vi "SensorReadOneLine.vi"() -> ()   [LabVIEW 2016]
uses:
  <vilib>/Instr/_visa.llb/VISA Configure Serial Port (Instr).vi
  Other Models/2010/Status/AxisDiagPacket.ctl
  Other Models/2010/Status/ControllerDiagPacket.ctl
  Control/Coordinate.ctl
panel:
  in  "file (use dialog)":path=path "C:/Users/TTUHEP/Documents/LabVIEW/output.txt"
  out "Boolean":bool=TRUE
  in  "baud rate":u32=115200
  in  "data bits":u16=8 min=5 max=8 step=1
  in  "parity":u16(ring)=2 items=["None", "Odd", "Even", "Mark", "Space"]
  in  "stop bits":u16(ring)=10 items=["1"=10, "1.5"=15, "2.0"=20]
  in  "flow control":u16(ring) items=["None"=0, "XON/XOFF"=1, "RTS/CTS"=2, "DTR/DSR"=4]
  in  "VISA resource name":refnum<visa-resource-name>="COM4"
  in  "Speed":dbl format="%#_13g"
  in  "EndPoint":T1 {"X" format="%#.5g"; "Y" format="%#.5g"; "Z" format="%#.6g"}
  in  "StartPoint":T1 {"X" format="%#.5g"; "Y" format="%#.5g"; "Z" format="%#.5g"}
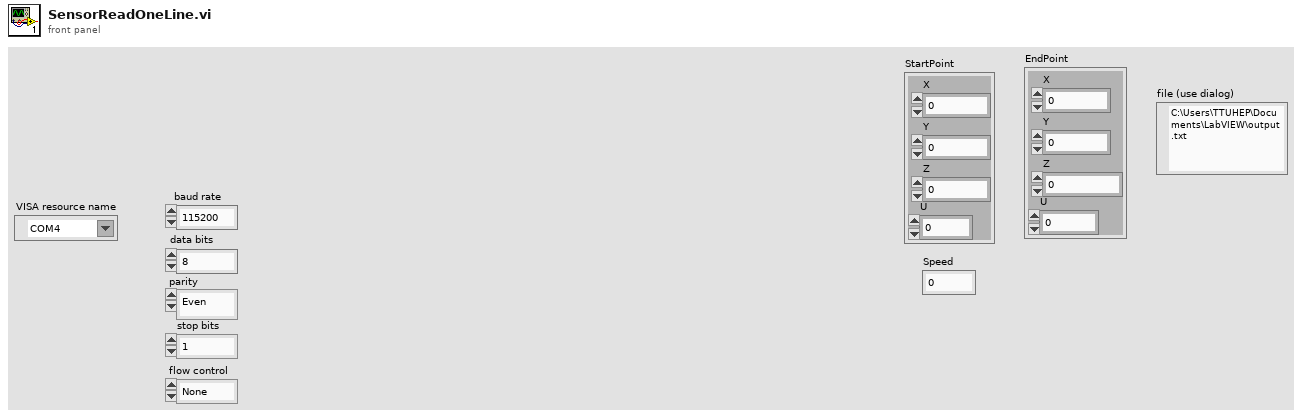
[diagram p1: front panel]
types:
  T1 = typedef "Coordinate.ctl" = cluster{"X":dbl, "Y":dbl, "Z":dbl, "U":dbl}
  T2 = typedef "ControllerDiagPacket.ctl" = cluster{"Number of Diag Packets":i32, "Axes":T3[], "error":errorcluster}
  T3 = typedef "AxisDiagPacket.ctl" = cluster{"Axis Name":string, "Analog Input 0":dbl, "Analog Input 1":dbl, "Axis Fault (num)":i32, "Axis Fault (str)":string, "Axis Fault (bits)":cluster{"AmplifierFault":bool, "AmplifierTemperatureFault":bool, "CcwEndOfTravelLimitFault":bool, "CcwSoftwareLimitFault":bool, "CommunicationLostFault":bool, "CwEndOfTravelLimitFault":bool, "CwSoftwareLimitFault":bool, "EmergencyStopFault":bool, "EncoderFault":bool, "ExternalFault":bool, "FeedbackScalingFault":bool, "GantryMisalignFault ":bool, "HallSensorFault":bool, "InPositionTimeoutFault":bool, "InternalFault":bool, "MarkerSearchFault":bool, "MaxVelocityCommandFault":bool, "MissedInterruptFault":bool, "MotorTemperatureFault":bool, "None":bool, "OverCurrentFault":bool, "PositionErrorFault":bool, "PositionFeedbackFault":bool, "PowerSupplyFault":bool, "ProbeInputFault":bool, "SafeZoneFault":bool, "VelocityErrorFault":bool, "VelocityFeedbackFault":bool, "VoltageClampFault":bool}, "Axis Status (num)":i32, "Axis Status (str)":string, "Axis Status (bits)":cluster{"BacklashActive":bool, "CalibrationEnabled1D":bool, "CalibrationEnabled2D":bool, "CommandValid":bool, "DriveAbortPending":bool, "DrivePending":bool, "Enabling":bool, "GainMappingEnabled":bool, "GantryAligned":bool, "GantryRealigning":bool, "Homed":bool, "Homing":bool, "IFOVEnabled":bool, "JogGenerating":bool, "Jogging":bool, "JoystickControl":bool, "MasterSlaveControl":bool, "MotionBlocked":bool, "MotionClamped":bool, "MoveDone":bool, "None":bool, "NotVirtual":bool, "Profiling":bool, "Stability0":bool, "Stability1":bool, "TrajectoryFiltering":bool, "WaitDone":bool}, "Current Command":sgl, "Current Error":sgl, "Current Feedback":sgl, "Digital Inputs":i32, "Digital Outputs":i32, "Drive Status":i32, "Drive Status (str)":string, "Drive Status (bits)":cluster{"AccelerationPhase":bool, "AutofocusActive":bool, "BrakeOutput":bool, "CcwEndOfTravelLimitInput":bool, "CosineEncoderError":bool, "CurrentClamp":bool, "CwEndOfTravelLimitInput":bool, "DecelerationPhase":bool, "DualLoopActive":bool, "EmergencyStopInput":bool, "Enabled":bool, "EncoderClipping":bool, "GalvoCalibrationEnabled":bool, "GalvoPowerCorrection":bool, "HallAInput":bool, "HallBInput":bool, "HallCInput":bool, "HighResolutionMode":bool, "HomeLimitInput":bool, "InPosition":bool, "InPosition2":bool, "MarkerInput":bool, "MarkerLatch":bool, "MoveActive":bool, "NoMotorSupply":bool, "None":bool, "PowerLimiting":bool, "ProgrammingFlash":bool, "ProgrammingMXH":bool, "PSOHaltLatch":bool, "ServoControl":bool, "SineEncoderError":bool}, "Position Feedback Auxiliary":dbl, "Position Command":dbl, "Position Error":dbl, "Position Feedback":dbl, "Program Position Command":dbl, "Program Position Error":dbl, "Program Position Feedback":dbl, "Velocity Command":dbl, "Velocity Error":dbl, "Velocity Feedback":dbl}
  T4 = cluster{"ControllerDiagPacket":T2, "read buffer":string}
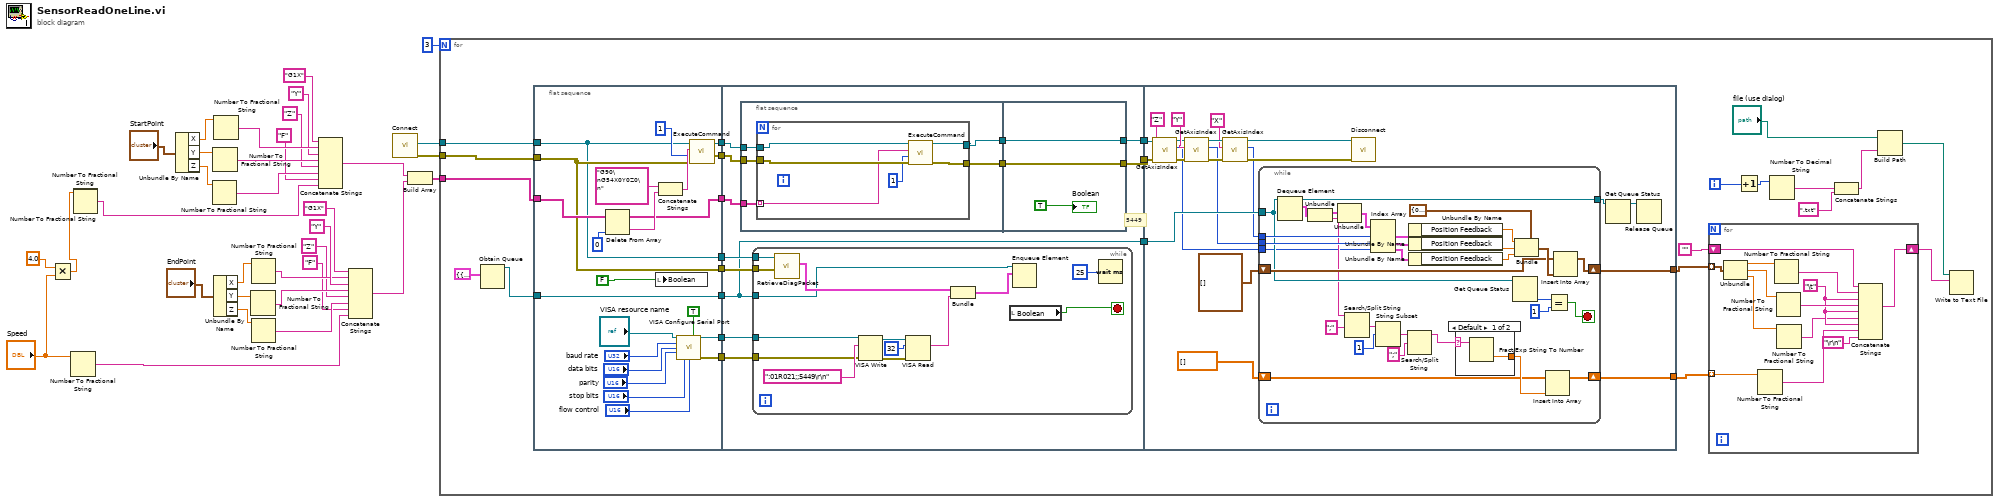
[diagram p0: block diagram]
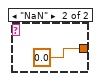
[diagram p2: hidden frame]
diagram:
  n1 = Multiply(x=4.0, y="Speed") -> (x*y=w2:dbl)
  n2 = Number To Fractional String(number="Speed") -> (F-format string=w8:string)  [unwired: 3 in]
  n3 = Number To Fractional String(number=w2) -> (F-format string=w1:string)  [unwired: 3 in]
  n4 = Number To Fractional String() -> ()  [unwired: 4 in, 1 out]
  n5 = Unbundle By Name("StartPoint") -> ("X"=w32:dbl, "Y"=w31:dbl, "Z"=w10:dbl)
  n6 = Number To Fractional String(number=w10) -> (F-format string=w15:string)  [unwired: 3 in]
  n7 = Number To Fractional String(number=w31) -> (F-format string=w29:string)  [unwired: 3 in]
  n8 = Number To Fractional String(number=w32) -> (F-format string=w30:string)  [unwired: 3 in]
  n9 = Unbundle By Name("EndPoint") -> ("X"=w21:dbl, "Y"=w22:dbl, "Z"=w13:dbl)
  n10 = Number To Fractional String(number=w22) -> (F-format string=w24:string)  [unwired: 3 in]
  n11 = Number To Fractional String(number=w21) -> (F-format string=w23:string)  [unwired: 3 in]
  n12 = Number To Fractional String(number=w13) -> (F-format string=w12:string)  [unwired: 3 in]
  n13 = Concatenate Strings("G1X", w30, "Y", w29, "Z", w15, "F", w1) -> (w19:string)
  n14 = Concatenate Strings("G1X", w23, "Y", w24, "Z", w12, "F", w8) -> (w18:string)
  n15 = call "Connect.vi"() -> ("error out"=w7:errorcluster, "controller"=w6:refnum<k24>)  [unwired: 10 in]
  n16 = Build Array(w19, w18) -> (w17:string[])
  n17 = for {
    N: 3 -> [_]
    tunnel: w17 -> [w49]
    tunnel: w7 -> [w42]
    tunnel: w6 -> [w41]
    i -> [w40]
    # "5449"
    n18 = Obtain Queue(element data type=cluster{"ControllerDiagPacket":T2, string} {"ControllerDiagPacket"={"Number of Diag Packets"=0, "Axes"=[], "error"={"status"=FALSE, "code"=0, "source"=""}}, ""}) -> (queue out=w47:refnum<queue>)  [unwired: 4 in, 2 out]
    n19 = flat-sequence {
      tunnel: [w89] -> w60
      tunnel: [w93] -> w59
      tunnel: [w94] -> w58
      tunnel: w49 -> [w95]
      tunnel: [w74] -> w57
      tunnel: [w75] -> w56
      tunnel: w47 -> [w87]
      tunnel: [w87] -> w55
      tunnel: [w79] -> w54
      tunnel: [w78] -> w53
      tunnel: w42 -> [w75]
      tunnel: w41 -> [w74]
      tunnel: [w102] -> w52
      tunnel: w60 -> [w96]
      tunnel: w59 -> [w98]
      tunnel: w58 -> [w97]
      tunnel: w57 -> [w106]
      tunnel: w56 -> [w107]
      tunnel: w55 -> [w105]
      tunnel: [w105] -> w51
      tunnel: w54 -> [w104]
      tunnel: w53 -> [w103]
      tunnel: [w99] -> w50
      tunnel: w52 -> [w141]
      tunnel: w51 -> [w156]
      tunnel: [w143] -> w43
      tunnel: [w142] -> w44
      tunnel: w50 -> [w140]
      frame #0 {
        n20 = Delete From Array(array=w95, index=0) -> (deleted portion=w90:string, array with subset deleted=w89:string[])  [unwired: 1 in]
        n21 = local write "Boolean"(FALSE) -> ()
        n22 = Concatenate Strings("G90\nG54X0Y0Z0\n", w90) -> (w88:string)
        n23 = call-poly "VISA Configure Serial Port"("VISA resource name"="VISA resource name", "Enable Termination\nChar (T)"=TRUE, "baud rate (9600)"="baud rate", "data bits (8)"="data bits", "parity (0:none)"="parity", "stop bits (10: 1 bit)"="stop bits", "flow control (0:none)"="flow control") -> ("VISA resource name out"=w79:refnum<visa-resource-name>, "error out"=w78:errorcluster)  [unwired: 7 in]
        n24 = call "ExecuteCommand.vi"("error in (no error)"=w75, "taskId"=1, "Command Code"=w88, "controller in"=w74) -> ("error out"=w94:errorcluster, "controller out"=w93:refnum<k24>)  [unwired: 5 in, 1 out]
      }
      frame #1 {
        n25 = flat-sequence {
          tunnel: [w112] -> w101
          tunnel: [w111] -> w100
          tunnel: w98 -> [w110]
          tunnel: w97 -> [w109]
          tunnel: w96 -> [w108]
          tunnel: [w120] -> w102
          tunnel: w101 -> [w120]
          tunnel: w100 -> [w119]
          tunnel: [w119] -> w99
          frame #0 {
            n26 = for {
              tunnel: w108 -> [w116] mode=indexing
              tunnel: w110 -> [w117]
              tunnel: w109 -> [w118]
              tunnel: [w114] -> w112
              tunnel: [w113] -> w111
              n27 = call "ExecuteCommand.vi"("error in (no error)"=w118, "taskId"=1, "Command Code"=w116, "controller in"=w117) -> ("error out"=w114:errorcluster, "controller out"=w113:refnum<k24>)  [unwired: 5 in, 1 out]
            }
          }
          frame #1 {
            "Boolean" <- TRUE
          }
        }
        n28 = while {
          tunnel: w106 -> [w135]
          tunnel: w107 -> [w134]
          tunnel: w105 -> [w122]
          tunnel: w104 -> [w131]
          tunnel: w103 -> [w129]
          stop <- w123 stop-if-true
          n29 = call "RetrieveDiagPacket.vi"("error in (no error)"=w134, "Controller In"=w135) -> ("ControllerDiagPacket"=w126:T2)  [unwired: 7 in, 2 out]
          n30 = VISA Write(VISA resource name=w131, write buffer=":01R021;;5449\r\n", error in (no error)=w129) -> (VISA resource name out=w132:refnum<visa-resource-name>, error out=w128:errorcluster)  [unwired: 1 out]
          n31 = VISA Read(VISA resource name=w132, byte count=u32 32, error in (no error)=w128) -> (read buffer=w125:string)  [unwired: 3 out]
          n32 = Bundle("ControllerDiagPacket"=w126, "read buffer"=w125) -> (w124:T4)  [unwired: 1 in]
          n33 = local read "Boolean"() -> (w123:bool)
          n34 = Enqueue Element(queue=w122, element=w124) -> ()  [unwired: 2 in, 3 out]
          n35 = Wait (ms)(milliseconds to wait=25) -> ()  [unwired: 1 out]
        }
      }
      frame #2 {
        n36 = call "GetAxisIndex.vi"("error in (no error)"=w141, "axis name"="Z", "controller in"=w140) -> ("error out"=w138:errorcluster, "axis index"=w136:i32, "controller out"=w139:refnum<k24>)  [unwired: 6 in]
        n37 = call "GetAxisIndex.vi"("error in (no error)"=w138, "axis name"="Y", "controller in"=w139) -> ("error out"=w154:errorcluster, "axis index"=w148:i32, "controller out"=w155:refnum<k24>)  [unwired: 6 in]
        n38 = call "GetAxisIndex.vi"("error in (no error)"=w154, "axis name"="X", "controller in"=w155) -> ("error out"=w153:errorcluster, "axis index"=w149:i32, "controller out"=w152:refnum<k24>)  [unwired: 6 in]
        n39 = while {
          tunnel: w149 -> [w186]
          tunnel: w148 -> [w185]
          shift-right: [w178] -> w142
          shift-left: cluster{"X":dbl, "Y":dbl, "Y 2":dbl}[] [] -> [w176]
          tunnel: [w177] -> w146
          tunnel: w156 -> [w172]
          shift-right: [w160] -> w143
          shift-left: dbl[] [] -> [w161]
          tunnel: w136 -> [w159]
          stop <- w174 stop-if-true
          n40 = Dequeue Element(queue=w172) -> (queue out=w177:refnum<queue>, element=w171:cluster{"ControllerDiagPacket":T2, string})  [unwired: 2 in, 2 out]
          n41 = Unbundle(w171) -> ("ControllerDiagPacket"=w170:T2, w164:string)
          n42 = Unbundle(w170) -> ("Axes"=w187:T3[])  [unwired: 2 out]
          n43 = Search/Split String(string=w164, search string/char (-)=";") -> (match + rest of string=w165:string)  [unwired: 1 in, 2 out]
          n44 = Index Array(array=w187, index #1=w186, index #2=w185, index #3=w159) -> (element #1=w184:T3, element #2=w183:T3, element #3=w158:T3)
          n45 = String Subset(string=w165, offset (0)=1) -> (substring=w167:string)  [unwired: 1 in]
          n46 = Search/Split String(string=w167, search string/char (-)=";") -> (substring before match=w163:string)  [unwired: 1 in, 2 out]
          n47 = Unbundle By Name(w184) -> ("Position Feedback"=w181:dbl)
          n48 = Unbundle By Name(w183) -> ("Position Feedback"=w180:dbl)
          n49 = Unbundle By Name(w158) -> ("Position Feedback"=w157:dbl)
          n50 = case shown="Default" w163 {
            selector: w163 -> [w189 _]
            tunnel: [w188 0.0] -> w162
            frame Default {
              n51 = Fract/Exp String To Number(string=w189) -> (number=w188:dbl)  [unwired: 3 in, 1 out]
            }
            frame "NaN" {
            }
          }
          n52 = Get Queue Status(queue=w172) -> (# elements in queue=w175:i32)  [unwired: 2 in, 7 out]
          n53 = Bundle(cluster=cluster{"X":dbl, "Y":dbl, "Z":dbl} {"X"=0.0, "Y"=0.0, "Z"=0.0}, "X"=w181, "Y"=w180, "Z"=w157) -> (w179:cluster{"X":dbl, "Y":dbl, "Z":dbl})
          n54 = Insert Into Array(array=w161, new element=w162) -> (w160:dbl[])  [unwired: 1 in]
          n55 = Equal?(x=w175, y=1) -> (x = y?=w174:bool)
          n56 = Insert Into Array(array=w176, new element=w179) -> (w178:cluster{"X":dbl, "Y":dbl, "Y 2":dbl}[])  [unwired: 1 in]
        }
        n57 = call "Disconnect.vi"("error in (no error)"=w153, "controller"=w152) -> ()  [unwired: 9 in, 1 out]
        n58 = Get Queue Status(queue=w146) -> (queue out=w145:refnum<queue>)  [unwired: 2 in, 7 out]
        n59 = Release Queue(queue=w145) -> ()  [unwired: 2 in, 3 out]
      }
    }
    n60 = for {
      tunnel: w44 -> [w73] mode=indexing
      tunnel: w43 -> [w70] mode=indexing
      shift-right: [w66] -> w46
      shift-left: "" -> [w67]
      w65 = "\t"
      n61 = Unbundle(w73) -> ("X"=w72:dbl, "Y"=w71:dbl, "Y 2"=w64:dbl)
      n62 = Number To Fractional String(number=w70) -> (F-format string=w62:string)  [unwired: 3 in]
      n63 = Number To Fractional String(number=w72) -> (F-format string=w69:string)  [unwired: 3 in]
      n64 = Number To Fractional String(number=w71) -> (F-format string=w68:string)  [unwired: 3 in]
      n65 = Number To Fractional String(number=w64) -> (F-format string=w63:string)  [unwired: 3 in]
      n66 = Concatenate Strings(w67, w69, w65, w68, w65, w63, w65, w62, "\r\n") -> (w66:string)
    }
    n67 = Increment(x=w40) -> (x+1=w34:i32)
    n68 = Number To Decimal String(number=w34) -> (decimal integer string=w39:string)  [unwired: 1 in]
    n69 = Concatenate Strings(w39, ".txt") -> (w36:string)
    n70 = Build Path(base path="file (use dialog)", name or relative path=w36) -> (appended path=w35:path)
    n71 = Write to Text File(file (use dialog)=w35, text=w46) -> ()  [unwired: 2 in, 3 out]
  }
